vi "Assert True.vi"(4 "Execution time (s)":dbl=-1.0, 6 "error code (1)":i32=1, 7 "Label":string, 8 "error in":errorcluster, 11 "True?":bool) -> (0 "error out":errorcluster, 2 "Properties":refnum<class "Properties.Assert.lvclass">)   [LabVIEW 2021, in "Banana.Caraya.lvlib" / "Platano.CarayaTestSuite.lvclass"]
uses:
  Platano.CarayaTestSuite.lvclass
  Platano.CarayaTestSuite.lvclass/Platano.CarayaTestSuite.ctl
  <vilib>/addons/_JKI Toolkits/Caraya/classes/Assert/Assert.lvclass
  Bananas/Platano/Platano.lvclass
  Bananas/Banana/Banana.lvclass
  Bananas/Leaf/Leaf.lvclass
  Leaf.Properties.Assert/Leaf.Properties.Assert.lvclass
  C:/Repositories/LVOS/Bananas/lv-src/Banana.Caraya/Leaf.Properties/Leaf.Properties.lvclass
  C:/Repositories/LVOS/Bananas/lv-src/Bananas/Leaf.Assertion/Leaf.Assertion.lvclass
  C:/Repositories/LVOS/Bananas/lv-src/Bananas/Leaf/Leaf.lvclass
  C:/Repositories/LVOS/Bananas/lv-src/Banana.Caraya/Leaf.Properties.Assert/Leaf.Properties.Assert.lvclass
  Bananas/AssertTrue/AssertTrue.lvclass
  C:/Repositories/LVOS/Bananas/lv-src/Bananas/AssertTrue/AssertTrue.lvclass
  C:/Repositories/LVOS/Bananas/lv-src/Bananas/BananaPeel/BananaPeel.lvclass
  <vilib>/addons/_JKI Toolkits/Caraya/classes/Properties.Assert/Properties.Assert.lvclass
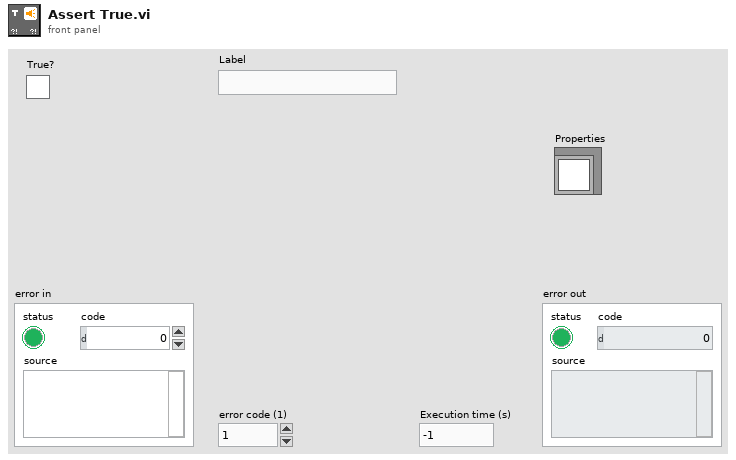
[diagram p1: front panel]
types:
  T1 = typedef "Bananas.lvlib/Assertion Strategies -- cluster.ctl" = cluster{"AssertTrue":refnum<class "AssertTrue.lvclass">, "AssertFalse":refnum<class "AssertFalse.lvclass">, "AssertEqualValue":refnum<class "AssertEqualValue.lvclass">, "AssertEqualType":refnum<class "AssertEqualType.lvclass">, "AssertCompareValue":refnum<class "AssertCompareValue.lvclass">, "AssertError":refnum<class "AssertError.lvclass">, "AssertAlmostEqual":refnum<class "AssertAlmostEqualValue.lvclass">}
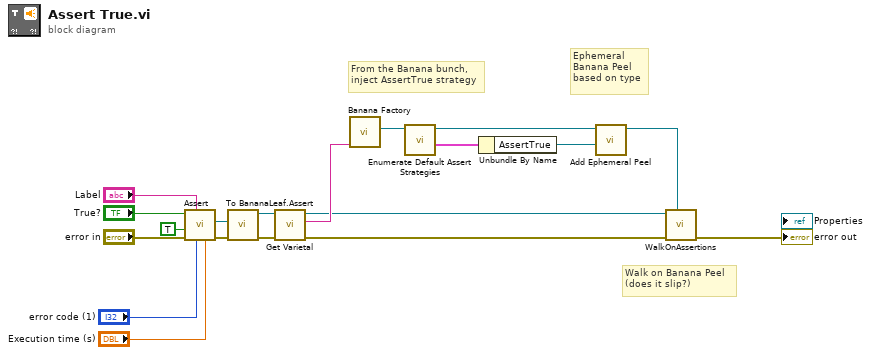
[diagram p0: block diagram]
diagram:
  # "Walk on Banana Peel\n(does it slip?)"
  # "From the Banana bunch,\ninject AssertTrue strategy"
  # "Ephemeral\nBanana Peel\nbased on type"
  n1 = call-poly <vilib>:"Assert.vi"("Execution time (s)"="Execution time (s)", "error code (1)"="error code (1)", "Label"="Label", "error in (no error)"="error in", "Register with caller test (F)"=TRUE, "True?"="True?") -> ("error out"=w5:errorcluster, "Properties"=w3:refnum<class "Properties.Assert.lvclass">)  [unwired: 4 in]
  n2 = call "To BananaLeaf.Assert.vi"("Properties.Assert"=w3) -> ("Leaf.Properties.Assert out"=w2:refnum<class "Leaf.Properties.Assert.lvclass">)  [unwired: 10 in]
  n3 = call "Get Varietal.vi"("error in (no error)"=w5, "Leaf in"=w2) -> ("error out"=w4:errorcluster, "Varietal"=w6:string, "Leaf out"=w1:refnum<class "Leaf.Properties.Assert.lvclass">)  [unwired: 7 in]
  n4 = call "Banana Factory.vi"("Varietal"=w6) -> ("Banana"=w7:refnum<class "Banana.lvclass">)  [unwired: 9 in, 1 out]
  n5 = call "Enumerate Default Assert Strategies.vi"("Banana"=w7) -> ("Strategies"=w8:T1, "Banana"=w9:refnum<class "Banana.lvclass">)  [unwired: 9 in]
  n6 = Unbundle By Name(w8) -> ("AssertTrue"=w10:refnum<class "AssertTrue.lvclass">)
  n7 = call "Add Ephemeral Peel.vi"("BananaPeel"=w10, "Banana"=w9) -> ("Banana"=w11:refnum<class "Banana.lvclass">)  [unwired: 9 in]
  n8 = call "WalkOnAssertions.vi"("Banana"=w11, "error in (no error)"=w4, "Leaf.Assertion"=w1) -> ("error out"=→"error out":errorcluster)  [unwired: 7 in, 1 out]
